vi "SlackAPI-users.identity.vi"(0 "token":string, 11 "error in (no error)":errorcluster) -> (4 "user":T1, 15 "error out":errorcluster)   [LabVIEW 2020]
uses:
  Typedefs/Slack-User.ctl
  <vilib>/httpClient/POSTBuffer.vi
  <vilib>/httpClient/LabVIEWHTTPClient.lvlib
panel:
  out "body":string
  out "headers":string
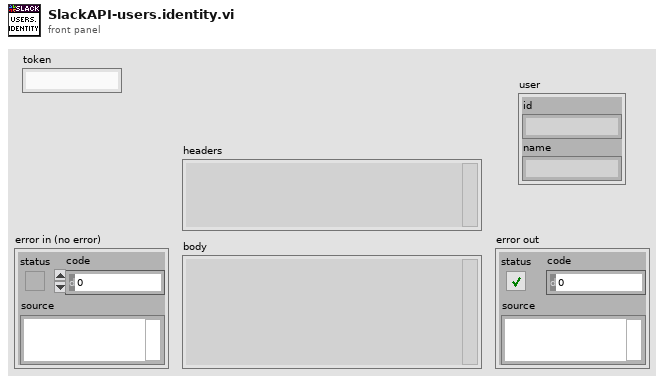
[diagram p1: front panel]
types:
  T1 = typedef "Slack-User.ctl" = cluster{"id":string, "name":string}
  T2 = typedef "LabVIEWHTTPClient.lvlib/ClientHandle.ctl" = refnum<k1>
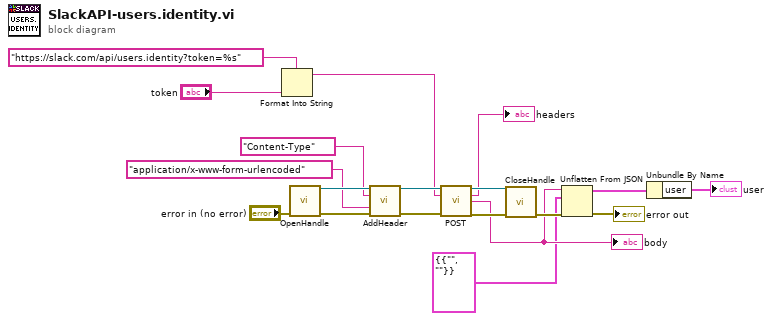
[diagram p0: block diagram]
diagram:
  n1 = Format Into String(format string="https://slack.com/api/users.identity?token=%s", "token") -> (resulting string=w12:string)  [unwired: 2 in, 1 out]
  n2 = call <vilib>:"OpenHandle.vi"("error in (no error)"="error in (no error)") -> ("client handle out"=w18:T2, "error out"=w19:errorcluster)  [unwired: 13 in]
  n3 = call <vilib>:"AddHeader.vi"("client handle"=w18, "header"="Content-Type", "value"="application/x-www-form-urlencoded", "error in (no error)"=w19) -> ("client handle out"=w14:T2, "error out"=w15:errorcluster)  [unwired: 10 in]
  n4 = call-poly <vilib>:"POST.vi"("client handle"=w14, "url"=w12, "error in (no error)"=w15) -> ("client handle out"=w11:T2, "headers"=→"headers":string, "body"=w4:string, "error out"=w10:errorcluster)  [unwired: 9 in]
  "body" <- w4
  n5 = call <vilib>:"CloseHandle.vi"("client handle"=w11, "error in (no error)"=w10) -> ("error out"=w6:errorcluster)  [unwired: 13 in]
  n6 = Unflatten From JSON(JSON string=w4, type and defaults=cluster{"user":T1} {"user"={"id"="", "name"=""}}, error in (no error)=w6) -> (value=w2:cluster{"user":T1}, error out=→"error out":errorcluster)  [unwired: 4 in]
  n7 = Unbundle By Name(w2) -> ("user"=→"user":T1)
